vi "AlliGator Update Settings Python Options.vi"(8 "error in (no error)":errorcluster, 11 "Python Settings Refnum":refnum<vi>) -> (0 "error out":errorcluster)   [LabVIEW 2021, in "AlliGator Settings.lvlib"]
doc: "Updates Python Plugins options in the Settings window."
uses:
  AlliGator Settings.lvlib
  AlliGator Python Settings.ctl
panel:
  in  "Python Settings":T1
  # "see the AlliGator License on the block diagram (Ctrl+E or Window:Show Block Diagram)"
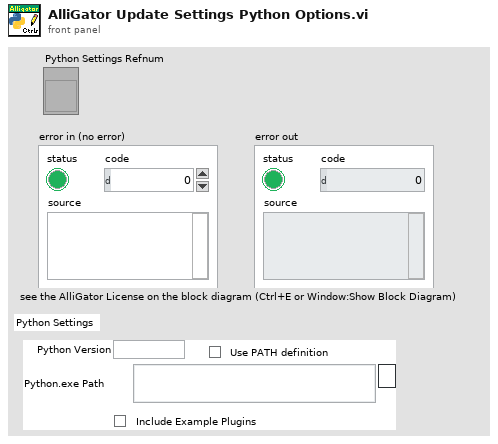
[diagram p1: front panel]
types:
  T1 = typedef "AlliGator Settings.lvlib/AlliGator Python Settings.ctl" = cluster{"Python Version":string, "Use PATH definition":bool, "Python.exe Path":path, "Include Example Plugins":bool}
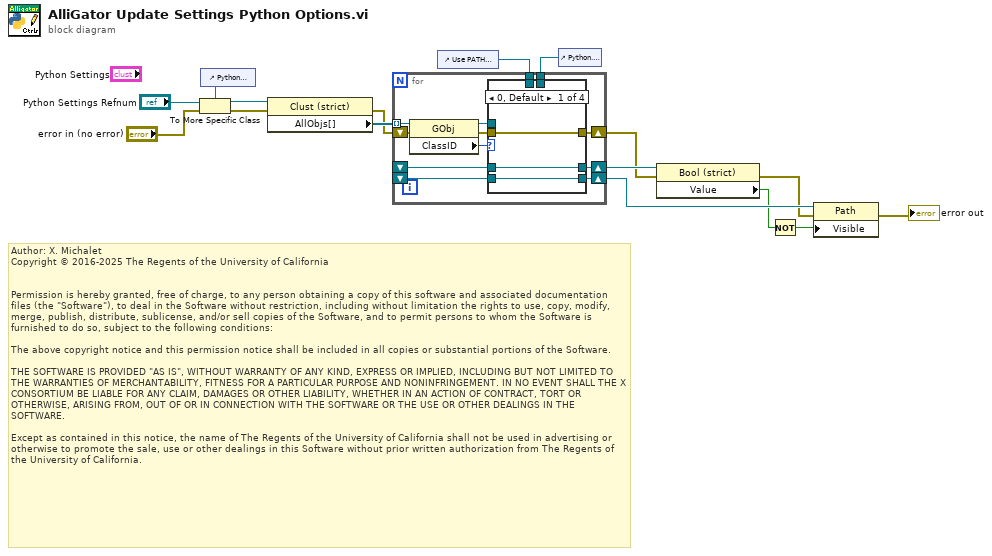
[diagram p0: block diagram]
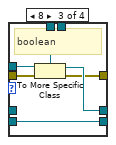
[diagram p3: hidden frame]
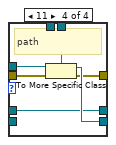
[diagram p4: hidden frame]
diagram:
  # "Author: X. Michalet\nCopyright © 2016-2025 The Regents of the University of California\n \n\nPermission is hereby granted, free of charge, to any person obtaining a copy of this software and associated documentation files (the \"Software\"), to deal in the Software without restriction, including without limitation the rights to use, copy, modify, merge, publish, distribute, sublicense, and/or sell copies of the Software, and to permit persons to whom the Software is furnished to do so, subject to the following conditions:\n\nThe above copyright notice and this permission notice shall be included in all copies or substantial portions of the Software.\n\nTHE SOFTWARE IS PROVIDED \"AS IS\", WITHOUT WARRANTY OF ANY KIND, EXPRESS OR IMPLIED, INCLUDING BUT NOT LIMITED TO THE WARRANTIES OF MERCHANTABILITY, FITNESS FOR A PARTICULAR PURPOSE AND NONINFRINGEMENT. IN NO EVENT SHALL THE X CONSORTIUM BE LIABLE FOR ANY CLAIM, DAMAGES OR OTHER LIABILITY, WHETHER IN AN ACTION OF CONTRACT, TORT OR OTHERWISE, ARISING FROM, OUT OF OR IN CONNECTION WITH THE SOFTWARE OR THE USE OR OTHER DEALINGS IN THE SOFTWARE.\n\nExcept as contained in this notice, the name of The Regents of the University of California shall not be used in advertising or otherwise to promote the sale, use or other dealings in this Software without prior written authorization from The Regents of the University of California."
  n1 = control-ref of="Python Settings"() -> (w13:refnum<vi>)
  n2 = To More Specific Class(target class=w13, reference="Python Settings Refnum", error in="error in (no error)") -> (specific class reference=w14:refnum<vi>, error out=w16:errorcluster)
  n3 = property class="Clust (strict)"(reference=w14, error in=w16) -> (error out=w10:errorcluster, "AllObjs[]"=w11:refnum<vi>[])  [unwired: 1 out]
  n4 = control-ref of="Use PATH definition"() -> (w8:refnum<vi>)
  n5 = control-ref of="Python.exe Path"() -> (w5:refnum<vi>)
  n6 = for {
    tunnel: w11 -> [w28] mode=indexing
    tunnel: w8 -> [w23]
    shift-right: [w24] -> w9
    shift-left: _ -> [w21]
    shift-right: [w18] -> w6
    shift-left: w10 -> [w25]
    shift-right: [w22] -> w7
    shift-left: _ -> [w20]
    tunnel: w5 -> [w17]
    n7 = property class="GObj"(reference=w28, error in=w25) -> (reference out=w26:refnum<vi>, error out=w19:errorcluster, "ClassID"=w27:u32)
    n8 = case shown="0, Default" w27 {
      tunnel: w26 -> [_ _ w39 w44]
      tunnel: [w31 w34 w40 w43] -> w24
      tunnel: w23 -> [_ _ w38 _]
      tunnel: [w30 w33 w36 w46] -> w22
      tunnel: w21 -> [w31 w34 _ w43]
      tunnel: w20 -> [w30 w33 w36 _]
      tunnel: w19 -> [w29 w32 w37 w45]
      tunnel: [w29 w32 w35 w42] -> w18
      tunnel: w17 -> [_ _ _ w41]
      frame 0, Default {
      }
      frame 27 {
        # "string"
      }
      frame 8 {
        # "boolean"
        n9 = To More Specific Class(target class=w38, reference=w39, error in=w37) -> (specific class reference=w40:refnum<vi>, error out=w35:errorcluster)
      }
      frame 11 {
        # "path"
        n10 = To More Specific Class(target class=w41, reference=w44, error in=w45) -> (specific class reference=w46:refnum<vi>, error out=w42:errorcluster)
      }
    }
  }
  n11 = property class="Bool (strict)"(reference=w9, error in=w6) -> (error out=w2:errorcluster, "Value"=w4:bool)  [unwired: 1 out]
  n12 = Not(x=w4) -> (.not. x?=w3:bool)
  n13 = property class="Path"(reference=w7, error in=w2, "Visible"=w3) -> (error out=→"error out":errorcluster)  [unwired: 1 out]
